vi "Chck MTCDT AP Slot Tests.vi"(6 "VISA resource  inname":refnum<visa-resource-name>="COM5", 7 "Passed so far?":bool, 8 "error in (no error)":errorcluster) -> (0 "error out":errorcluster, 4 "Visa resource name out":refnum<visa-resource-name>, 5 "All Passed?":bool)   [LabVIEW 2024]
uses:
  AP slots to test.ctl
panel:
  in  "Slot":T1=enum."AP1 and AP2"
  in  "Start":bool
  out "Test Log":string
  # "MTCDT AP Slot Tests"
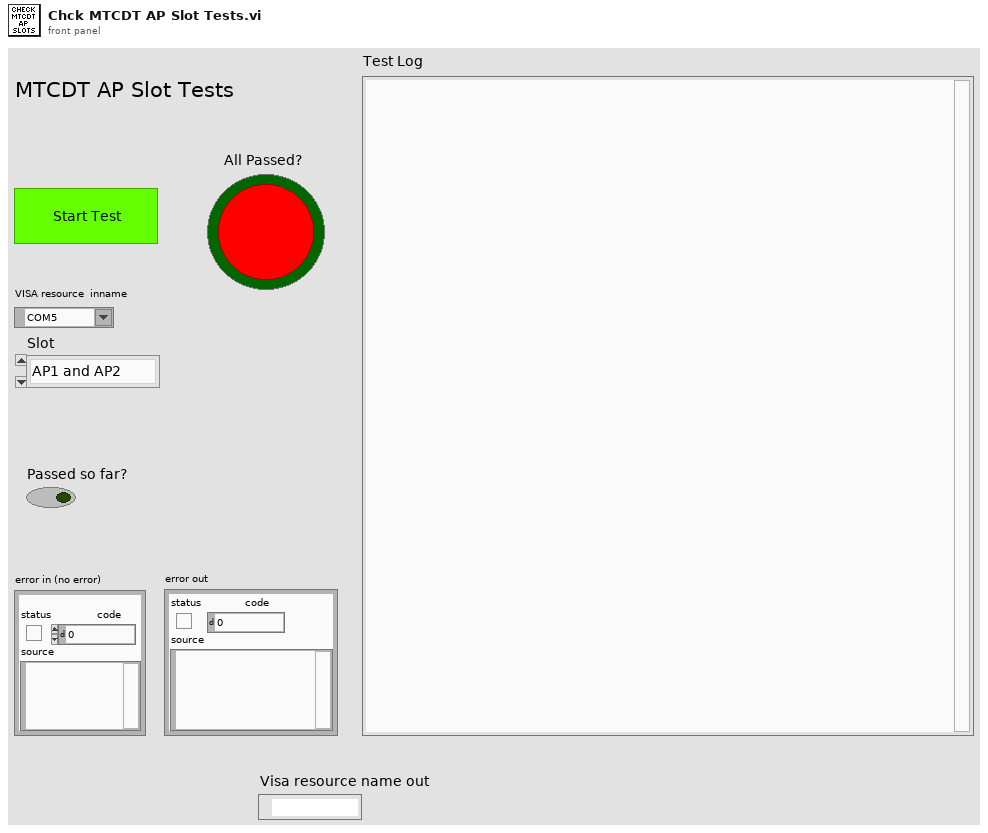
[diagram p1: front panel]
types:
  T1 = typedef "AP slots to test.ctl" = enum16{"Select Slot", "AP1", "AP2", "AP1 and AP2"}
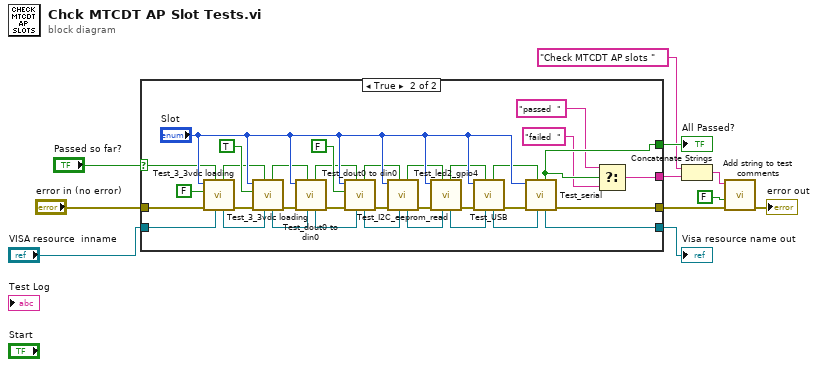
[diagram p0: block diagram]
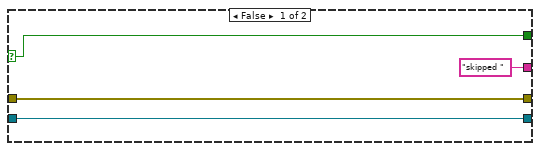
[diagram p2: hidden frame]
diagram:
  n1 = case shown="True" "Passed so far?" {
    selector: "Passed so far?" -> [w14 w48]
    tunnel: "VISA resource  inname" -> [w15 w47]
    tunnel: [w15 w46] -> w9
    tunnel: [w14 w45] -> w8
    tunnel: [w12 w44] -> w6
    tunnel: ["skipped " w41] -> w2
    tunnel: "error in (no error)" -> [w12 w16]
    frame False {
    }
    frame True {
      n2 = call "Test_3_3vdc loading.vi"("VISA resource name"=w47, "Pass so far?"=w48, "error in (no error)"=w16, "3.3vdc Load ON (y)"=FALSE, "Slot"="Slot") -> ("error out"=w30:errorcluster, "VISA resource name out"=w27:refnum<visa-resource-name>, "Passed?"=w29:bool)  [unwired: 2 in, 2 out]
      n3 = call "Test_3_3vdc loading.vi"("VISA resource name"=w27, "Pass so far?"=w29, "error in (no error)"=w30, "3.3vdc Load ON (y)"=TRUE, "Slot"="Slot") -> ("error out"=w25:errorcluster, "VISA resource name out"=w26:refnum<visa-resource-name>, "Passed?"=w28:bool)  [unwired: 2 in, 2 out]
      n4 = call "Test_dout0 to din0.vi"("VISA resource name"=w26, "Passed so far?"=w28, "error in (no error)"=w25, "Slot"="Slot") -> ("error out"=w40:errorcluster, "VISA resource name out"=w37:refnum<visa-resource-name>, "Passed?"=w38:bool)  [unwired: 4 in, 1 out]
      n5 = call "Test_dout0 to din0.vi"("VISA resource name"=w37, "Passed so far?"=w38, "error in (no error)"=w40, "Dout0 ON (y)"=FALSE, "Slot"="Slot") -> ("error out"=w36:errorcluster, "VISA resource name out"=w34:refnum<visa-resource-name>, "Passed?"=w35:bool)  [unwired: 3 in, 1 out]
      n6 = call "Test_I2C_eeprom_read.vi"("VISA resource name"=w34, "Passed so far?"=w35, "error in (no error)"=w36, "Slot"="Slot") -> ("error out"=w33:errorcluster, "VISA resource name out"=w32:refnum<visa-resource-name>, "Passed?"=w20:bool)  [unwired: 4 in, 1 out]
      n7 = call "Test_led2_gpio4.vi"("VISA resource name"=w32, "Passed so far?"=w20, "error in (no error)"=w33, "Slot"="Slot") -> ("error out"=w24:errorcluster, "VISA resource name out"=w23:refnum<visa-resource-name>, "Passed?"=w18:bool)  [unwired: 4 in, 1 out]
      n8 = call "Test_USB.vi"("VISA resource name"=w23, "Passed so far?"=w18, "error in (no error)"=w24, "Slot"="Slot") -> ("error out"=w22:errorcluster, "VISA resource name out"=w21:refnum<visa-resource-name>, "Passed?"=w19:bool)  [unwired: 4 in, 1 out]
      n9 = call "Test_serial.vi"("VISA resource name"=w21, "Passed so far?"=w19, "error in (no error)"=w22, "Slot"="Slot") -> ("error out"=w44:errorcluster, "VISA resource name out"=w46:refnum<visa-resource-name>, "Passed?"=w45:bool)  [unwired: 4 in, 1 out]
      n10 = Select(t="passed  ", s=w45, f="failed  ") -> (s? t:f=w41:string)
    }
  }
  "Visa resource name out" <- w9
  "All Passed?" <- w8
  n11 = Concatenate Strings("Check MTCDT AP slots " ("Comments"), w2) -> (w1:string)
  n12 = call "Add string to test comments.vi"("error in (no error)"=w6, "New Section (y)?"=FALSE, "Comments"=w1) -> ("error out"=→"error out":errorcluster)  [unwired: 7 in, 1 out]
